vi "Read Data Timestamp.vi"(8 "error in (no error)":errorcluster, 11 "Data":refnum<class "Data.lvclass">) -> (0 "error out":errorcluster, 2 "timestamp":timestamp, 3 "Data":refnum<class "Data.lvclass">)   [LabVIEW 2017, in "Data.lvclass"]
uses:
  <vilib>/addons/_NISVFA/_Shared subVIs/Data Objects/Data/Data.lvclass
  <vilib>/addons/_NISVFA/_Shared subVIs/Data Objects/Data/Data.lvclass/Data.ctl
  <vilib>/addons/_NISVFA/_Shared subVIs/Common/sv_Get NI Property Name String.vi
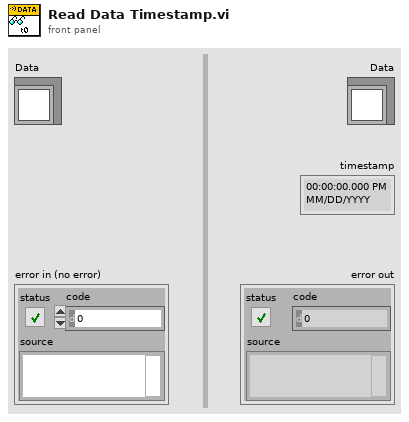
[diagram p1: front panel]
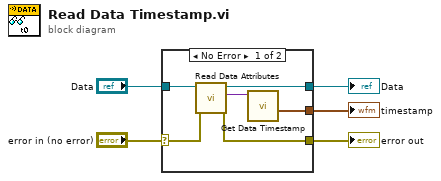
[diagram p0: block diagram]
diagram:
  n1 = case shown="No Error" "error in (no error)" {
    selector: "error in (no error)" -> [w7 w12]
    tunnel: "Data" -> [w11 w13]
    tunnel: [w10 w13] -> w4
    tunnel: [w6 _] -> w3
    tunnel: [w8 w12] -> w2
    frame No Error {
      n2 = call <vilib>:"Read Data Attributes.vi"("error in (no error)"=w7, "Data in"=w11) -> ("error out"=w8:errorcluster, "data attributes"=w9:variant, "Data out"=w10:refnum<class "Data.lvclass">)  [unwired: 7 in]
      n3 = call <vilib>:"Get Data Timestamp.vi"("variant in"=w9) -> ("timestamp"=w6:timestamp)  [unwired: 9 in, 1 out]
    }
    frame Error {
    }
  }
  "Data" <- w4
  "error out" <- w2
  "timestamp" <- w3
